vi "test Import Terminals.vi"(8 "error in":errorcluster, 11 "TestCase in":refnum<class "1553 Parameters Import.lvclass">) -> (0 "error out":errorcluster, 3 "TestCase out":refnum<class "1553 Parameters Import.lvclass">)   [LabVIEW 2020, in "1553 Parameters Import.lvclass"]
uses:
  1553 Parameters Import.lvclass
  Shared/Address.ctl
  1553 Parameters Import.lvclass/1553 Parameters Import.ctl
  <vilib>/addons/_JKI Toolkits/VI Tester/TestCase.llb/TestCase.lvclass
  C:/Program Files (x86)/National Instruments/LabVIEW 2020/vi.lib/addons/_JKI Toolkits/VI Tester/TestCase.llb/TestCase.lvclass
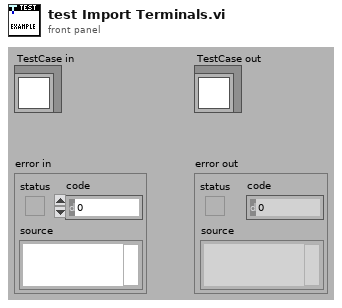
[diagram p1: front panel]
types:
  T1 = typedef "Address.ctl" = u16
  T2 = typedef "1553 Channel.ctl" = cluster{"HW channel":u16, "terminal addresses":T1[], "acyclic frame names":string[], "messages":T3[]}
  T3 = typedef "Message Definition.ctl" = cluster{"name":string, "message type":T4, "endpoint Tx":T5, "endpoint Rx":T5, "create timestamp channel":bool, "mode code":u16, "number of words":u16, "parameters":cluster{"name":string, "default value":dbl, "unit":string, "parameter definition":T6}[]}
  T4 = typedef "Message Type.ctl" = string
  T5 = typedef "Terminal Endpoint.ctl" = cluster{"terminal address":T1, "subaddress":T1}
  T6 = typedef "Parameter Definition.ctl" = cluster{"start index":i32, "size (bits)":i32, "encoding":enum16{"BNR", "BCD", "Discrete"}, "signed":bool, "multiplier":dbl, "offset":dbl}
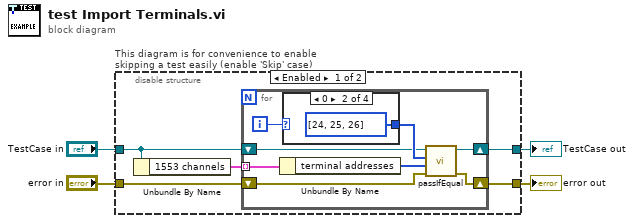
[diagram p0: block diagram]
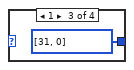
[diagram p3: hidden frame]
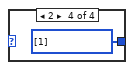
[diagram p4: hidden frame]
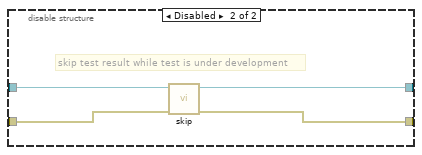
[diagram p5: hidden frame]
diagram:
  n1 = disable-structure "This diagram is for convenience to enable skipping a test easily (enable 'Skip' case)" shown="Enabled" {
    disable-tunnel: "TestCase in" -> [w9 w24]
    disable-tunnel: [w6 w22] -> w1
    disable-tunnel: [w5 w23] -> w3
    disable-tunnel: "error in" -> [w8 w21]
    frame Enabled {
      n2 = Unbundle By Name(w9) -> ("1553 channels"=w7:T2[])
      n3 = for {
        tunnel: w7 -> [w13] mode=indexing
        shift-right: [w11] -> w6
        shift-left: w9 -> [w15]
        shift-right: [w10] -> w5
        shift-left: w8 -> [w14]
        i -> [w12]
        n4 = Unbundle By Name(w13) -> ("terminal addresses"=w17:T1[])
        n5 = case shown="0" w12 {
          tunnel: [_ T1[] [24, 25, 26] ("terminals") T1[] [31, 0] ("terminals") T1[] [1] ("terminals")] -> w16
          frame Default {
          }
          frame 0 {
          }
          frame 1 {
          }
          frame 2 {
          }
        }
        n6 = call-dynamic "passIfEqual.vi"("error in (no error)"=w14, "y"=w17, "x"=w16, "TestCase in"=w15) -> ("error out"=w10:errorcluster, "TestCase out"=w11:refnum<class "1553 Parameters Import.lvclass">)  [unwired: 6 in]
      }
    }
    frame Disabled {
      # "skip test result while test is under development"
      n7 = call <vilib>:"skip.vi"("error in (no error)"=w21, "TestCase in"=w24) -> ("error out"=w23:errorcluster, "TestCase out"=w22:refnum<class "1553 Parameters Import.lvclass">)  [unwired: 8 in]
    }
  }
  "error out" <- w3
  "TestCase out" <- w1
